vi "SPI.vi"() -> ()   [LabVIEW 2019]
uses:
  <vilib>/myRIO/Instrument Drivers/Onboard IO/SPI/typedefs/SPI User Configuration.ctl
  <vilib>/myRIO/Common/Instrument Driver Framework/myRIO v1.0/SPI/typedefs/SPI Clock Phase.ctl
  <vilib>/myRIO/Common/Instrument Driver Framework/myRIO v1.0/SPI/typedefs/SPI Clock Polarity.ctl
  <vilib>/myRIO/Common/Instrument Driver Framework/myRIO v1.0/SPI/typedefs/SPI Data Direction.ctl
  <vilib>/myRIO/Common/Instrument Driver Framework/myRIO v1.0/SPI/typedefs/SPI Frame Length.ctl
  <vilib>/myRIO/Common/Instrument Driver Framework/myRIO v1.0/UART/vis/myRIO v1.0 Close UART.vi
  <vilib>/myRIO/Common/Instrument Driver Framework/ELVIS III v1.0/Resource Manager/vis/ELVIS III v1.0 Create Configuration List.vi
  <vilib>/Utility/error.llb/Error Cluster From Error Code.vi
  <vilib>/myRIO/Common/Instrument Driver Framework/ELVIS III v1.0/Resource Manager/vis/ELVIS III v1.0 Configure IO.vi
  <vilib>/myRIO/Common/Instrument Driver Framework/ELVIS III v1.0/Resource Manager/vis/ELVIS III v1.0 Unreserve Channel List.vi
  <vilib>/myRIO/Common/Instrument Driver Framework/myRIO v1.0/myRIO v1.0 Close.vi
  <vilib>/myRIO/Common/Instrument Driver Framework/Utilities/vis/FPGA Ref Manager.vi
  <vilib>/myRIO/Common/Instrument Driver Framework/ELVIS III v1.0/ELVIS III v1.0 Reset FPGA.vi
  <vilib>/myRIO/Common/Instrument Driver Framework/myRIO v1.0/IRQ/vis/myRIO v1.0 IRQ Info FGV.vi
  <vilib>/myRIO/Common/Instrument Driver Framework/myRIO v1.0/IRQ/vis/myRIO v1.0 Timer IRQ Info FGV.vi
  <vilib>/myRIO/Common/Instrument Driver Framework/myRIO v1.0/IRQ/vis/myRIO v1.0 ISR Agent.vi
  <vilib>/myRIO/Instrument Drivers/Utilities/vis/Reset Index.vi
  <vilib>/myRIO/Common/Instrument Driver Framework/myRIO v1.0/Resource Manager/vis/myRIO v1.0 Block Write Resource Manager.vi
  <vilib>/myRIO/Instrument Drivers/Utilities/Utilities.lvlib
  <vilib>/myRIO/Instrument Drivers/Onboard IO/SPI/SPI.lvlib
panel:
  out "Frames Read":u16[](array[numeric])
  in  "Frames to Write":u16[](array[numeric])=[3, 0, 4, 0, 0, 0, 0, 1]
  # "ELVIS III Control IO"
  # "SPI"
  # "Overview: Performs a simultaneous SPI Write/Read operation on the Bank A SPI lines (MISO: A/DIO6, MOSI: A/DIO7).\nInstructions:\n1. Connect a wire from A/DIO6 to A/DIO7.\n2. Change the values in Frames to Write.\n3. Run the VI.\n4. Notice Frames Read contains the same values written to Frames to Write."
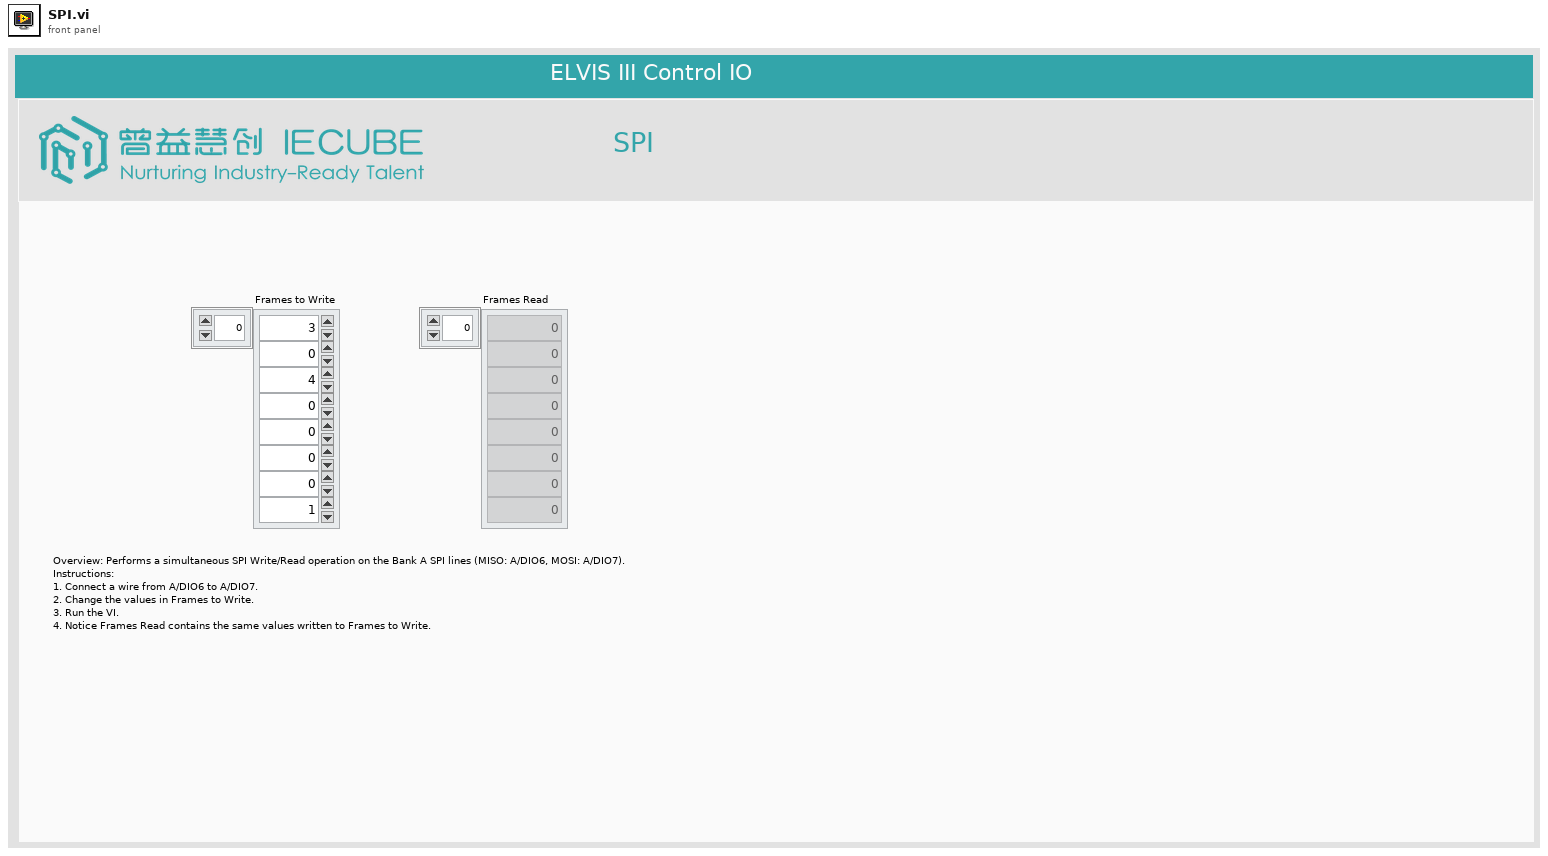
[diagram p1: front panel]
types:
  T1 = typedef "SPI.lvlib/SPI User Configuration.ctl" = cluster{"Frequency [Hz]":dbl, "Clock Phase":T2, "Clock Polarity":T3, "Data Direction":T4, "Frame Length":T5}
  T2 = typedef "SPI Clock Phase.ctl" = enum8{"Leading", "Trailing"}
  T3 = typedef "SPI Clock Polarity.ctl" = enum8{"Low", "High"}
  T4 = typedef "SPI Data Direction.ctl" = enum8{"Most significant bit first", "Least significant bit first"}
  T5 = typedef "SPI Frame Length.ctl" = u8
  T6 = typedef "SPI.lvlib/SPI Reference.ctl" = cluster{"myRIO Reference":T7, "SPI Channels Enum":T11, "SPI Configuration":T12}
  T7 = typedef "myRIO Generic Hardware Reference.ctl" = cluster{"myRIO Model":T8, "myRIO Hardware Reference":T9}
  T8 = typedef "Hardware Version Enum.ctl" = enum16{"Unknown", "myRIO-1900", "myRIO-1950", "roboRIO", "NI ELVIS RIO CM", "ELVIS III"}
  T9 = typedef "myRIO v1.0 Reference.ctl" = cluster{"Generic FPGA Reference":T10, "Allow multiple opens":bool}
  T10 = typedef "Generic FPGA Reference.ctl" = refnum<k20>
  T11 = typedef "SPI Channels Enum.ctl" = enum16{"Not Connected", "A/SPI", "B/SPI", "SPI/SPI"}
  T12 = typedef "SPI.lvlib/SPI Configuration.ctl" = cluster{"Frequency [Hz]":dbl, "Clock Phase":T2, "Clock Polarity":T3, "Data Direction":T4, "Frame Length":T5}
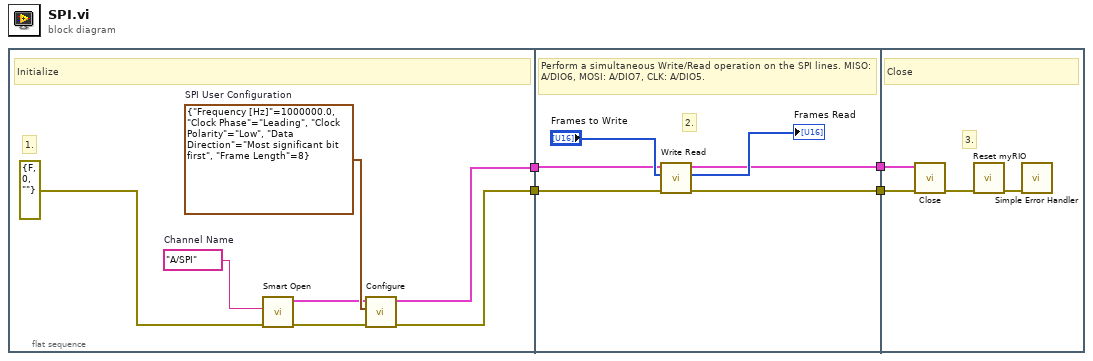
[diagram p0: block diagram]
diagram:
  n1 = flat-sequence {
    tunnel: [w6] -> w3
    tunnel: [w5] -> w2
    tunnel: [w16] -> w4
    tunnel: w3 -> [w17]
    tunnel: w2 -> [w13]
    tunnel: [w12] -> w1
    tunnel: w4 -> [w20]
    tunnel: w1 -> [w18]
    frame #0 {
      w11 = T1 {"Frequency [Hz]"=1000000.0, "Clock Phase"=enum."Leading", "Clock Polarity"=enum."Low", "Data Direction"=enum."Most significant bit first", "Frame Length"=8}  # SPI User Configuration
      w10 = tag "A/SPI"  # Channel Name
      # "1."
      # "Initialize"
      n2 = call <vilib>:"Smart Open.vi"("error in (no error)"=errorcluster {"status"=FALSE, "code"=0, "source"=""} ("Error In"), "Channel Name"=w10) -> ("error out"=w7:errorcluster, "SPI Ref Out"=w8:T6)  [unwired: 8 in]
      n3 = call <vilib>:"Configure.vi"("error in (no error)"=w7, "SPI User Configuration"=w11, "SPI Ref In"=w8) -> ("error out"=w6:errorcluster, "SPI Ref Out"=w5:T6)  [unwired: 7 in]
    }
    frame #1 {
      # "2."
      # "Perform a simultaneous Write/Read operation on the SPI lines. MISO: A/DIO6, MOSI: A/DIO7, CLK: A/DIO5."
      n4 = call <vilib>:"Write Read.vi"("error in (no error)"=w17, "Frames to Write"="Frames to Write", "SPI Ref In"=w13) -> ("error out"=w16:errorcluster, "Frames Read"=→"Frames Read":u16[], "SPI Ref Out"=w12:T6)  [unwired: 6 in]
    }
    frame #2 {
      # "3."
      # "Close"
      n5 = call <vilib>:"Close.vi"("error in (no error)"=w20, "SPI Ref In"=w18) -> ("error out"=w19:errorcluster)  [unwired: 9 in]
      n6 = call <vilib>:"Reset myRIO.vi"("error in (no error)"=w19) -> ("error out"=w21:errorcluster)  [unwired: 10 in]
      n7 = call <vilib>:"Simple Error Handler.vi"("error in (no error)"=w21) -> ()  [unwired: 4 in, 5 out]
    }
  }
